vi "DIO64 Close.vi"(0 "board in":u16 format="%.0x", 11 "error in (no error)":errorcluster) -> (4 "board out":u16 format="%.0x", 15 "error out":errorcluster)   [LabVIEW 2012]
doc: "This VI closes the connection to the selected digital I/O board.\n\nCopyright (c) 2002 Viewpoint Systems Inc. All Rights Reserved"
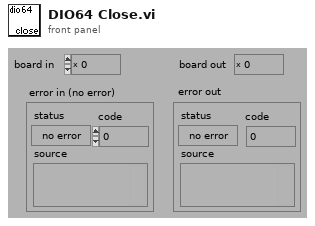
[diagram p1: front panel]
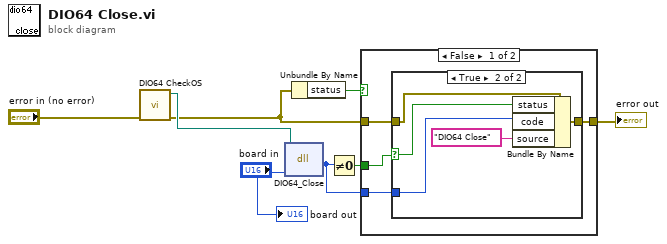
[diagram p0: block diagram]
diagram:
  n1 = call "DIO64 CheckOS.vi"("error in"="error in (no error)") -> ("error out"=w1:errorcluster, "path in"=w3:path)  [unwired: 9 in]
  n2 = dll-call lib="C:/DIO64Visa/DLL/DIO64_Visa32/Debug/DIO64_Visa32.dll" fn="DIO64_Close"(path in=w3, "board"="board in") -> ("return type"=w4:i32)  [unwired: 3 in, 2 out]
  n3 = Unbundle By Name(w1) -> ("status"=w8:bool)
  n4 = Not Equal To 0?(x=w4) -> (x != 0?=w6:bool)
  n5 = case shown="False" w8 {
    tunnel: w1 -> [w10 w19]
    tunnel: [w12 w19] -> w5
    tunnel: w6 -> [w11 _]
    tunnel: w4 -> [w9 _]
    frame False {
      n6 = case shown="True" w11 {
        selector: w11 -> [_ w16]
        tunnel: [w13 w17] -> w12
        tunnel: w10 -> [w13 w14]
        tunnel: w9 -> [_ w15]
        frame False {
        }
        frame True {
          n7 = Bundle By Name(cluster=w14, "status"=w16, "code"=w15, "source"="DIO64 Close") -> (w17:errorcluster)
        }
      }
    }
    frame True {
    }
  }
  "error out" <- w5
  "board out" <- "board in"
